vi "Get Count.vi"(8 "error in (no error)":errorcluster, 11 "Core Threads Configuration in":refnum<class "Core Threads Configuration.lvclass">) -> (0 "error out":errorcluster, 2 "count":i32, 3 "Core Threads Configuration out":refnum<class "Core Threads Configuration.lvclass">)   [LabVIEW 2017, in "DSF Core.lvlib" / "Core Threads Configuration.lvclass"]
uses:
  Core Threads Configuration.lvclass
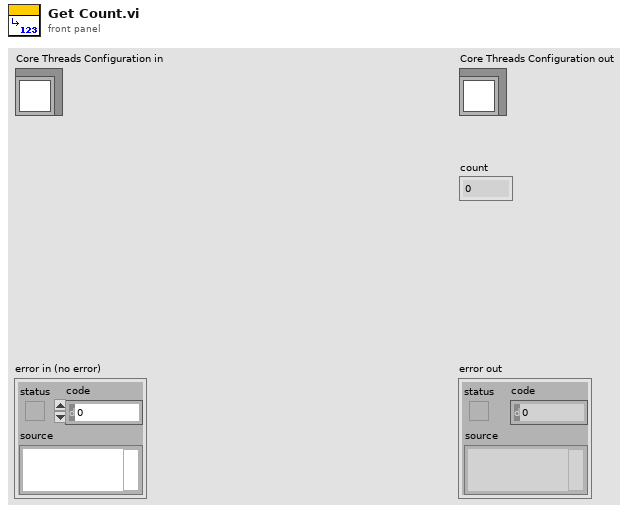
[diagram p1: front panel]
types:
  T1 = typedef "DSF Core.lvlib/Core Threads Configuration.lvclass/Configuration.ctl" = cluster{"processor":i32, "priority offset":i16}
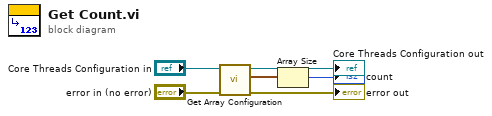
[diagram p0: block diagram]
diagram:
  n1 = call "Get Array Configuration.vi"("error in (no error)"="error in (no error)", "Core Threads Configuration in"="Core Threads Configuration in") -> ("error out"=→"error out":errorcluster, "thread configurations"=w3:T1[], "Core Threads Configuration out"=→"Core Threads Configuration out":refnum<class "Core Threads Configuration.lvclass">)  [unwired: 7 in]
  n2 = Array Size(array=w3) -> (size(s)=→"count":i32)
